vi "pythonHyperstackTest.vi"() -> ()   [LabVIEW 2017]
uses:
  globalUtilities.vi
panel:
  out "optogGUIX":dbl
  out "optogGUIY":dbl
  out "optogGUIZ":dbl
  out "return":dbl
  in  "stop":bool
  # "Arrays work only if they have size >1 (2 is fine). Dunno why."
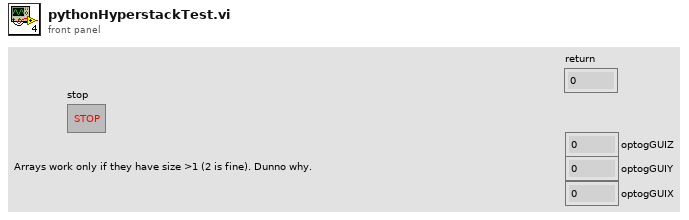
[diagram p1: front panel]
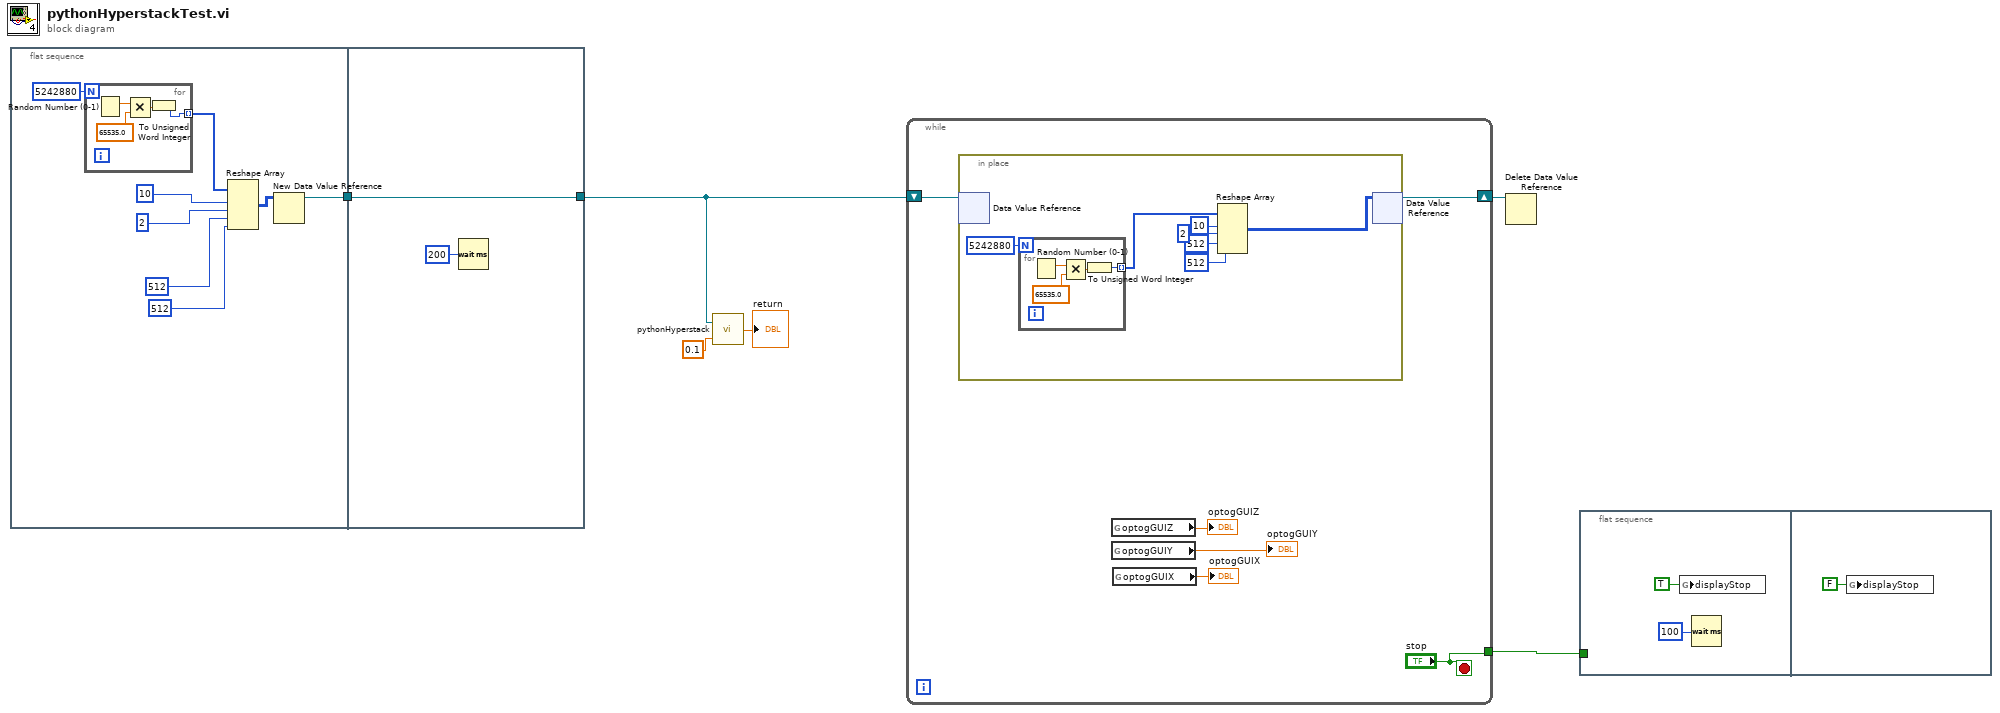
[diagram p0: block diagram]
diagram:
  n1 = flat-sequence {
    tunnel: [w11] -> w4
    tunnel: [w20] -> w2
    tunnel: w4 -> [w20]
    frame #0 {
      n2 = for {
        N: 5242880 ("dimension size") -> [_]
        tunnel: [w15] -> w13 mode=indexing
        n3 = Random Number (0-1)() -> (number: 0 to 1=w18:dbl)
        n4 = Multiply(x=w18, y=65535.0) -> (x*y=w16:dbl)
        n5 = To Unsigned Word Integer(number=w16) -> (unsigned 16bit integer=w15:u16)
      }
      n6 = Reshape Array(w13, 10 ("dimension size"), 2 ("dimension size"), 512 ("dimension size"), 512 ("dimension size")) -> (w12:u16[][][][])
      n7 = New Data Value Reference(data value=w12) -> (data value reference=w11:refnum<data-value>)  [unwired: 1 in, 1 out]
    }
    frame #1 {
      n8 = Wait (ms)(milliseconds to wait=u32 200) -> ()  [unwired: 1 out]
    }
  }
  n9 = call "pythonHyperstack.vi"("refresh_time"=0.1, "image reference"=w2) -> ("return type"=→"return":dbl)
  n10 = while {
    tunnel: ["stop"] -> w5
    shift-right: [w25] -> w6
    shift-left: w2 -> [w26]
    stop <- "stop" stop-if-true
    n11 = in-place {
      n12 = in-place-dvr #1(w26) -> ()  [unwired: 2 out]
      n13 = for {
        N: 5242880 ("dimension size") -> [_]
        tunnel: [w37] -> w32 mode=indexing
        n14 = Random Number (0-1)() -> (number: 0 to 1=w36:dbl)
        n15 = Multiply(x=w36, y=65535.0) -> (x*y=w34:dbl)
        n16 = To Unsigned Word Integer(number=w34) -> (unsigned 16bit integer=w37:u16)
      }
      n17 = Reshape Array(w32, 10 ("dimension size"), 2 ("dimension size"), 512 ("dimension size"), 512 ("dimension size")) -> (w31:u16[][][][])
      n18 = in-place-dvr #1(w31) -> (w25:refnum<data-value>)  [unwired: 1 out]
    }
    n19 = global read "globalUtilities.vi" "optogGUIZ"() -> (→"optogGUIZ":dbl)
    n20 = global read "globalUtilities.vi" "optogGUIY"() -> (→"optogGUIY":dbl)
    n21 = global read "globalUtilities.vi" "optogGUIX"() -> (→"optogGUIX":dbl)
  }
  n22 = Delete Data Value Reference(data value reference=w6) -> ()  [unwired: 1 in, 2 out]
  n23 = flat-sequence {
    tunnel: w5 -> [_]
    frame #0 {
      n24 = global write "globalUtilities.vi" "displayStop"(TRUE ("generalStop")) -> ()
      n25 = Wait (ms)(milliseconds to wait=u32 100) -> ()  [unwired: 1 out]
    }
    frame #1 {
      n26 = global write "globalUtilities.vi" "displayStop"(FALSE ("generalStop")) -> ()
    }
  }
